vi "read1Byte Tx Rx.vi"(7 "address":u16, 8 "error in (no error)":errorcluster, 9 "id":u8, 10 "protocol_version":i32, 11 "port_num":i32) -> (0 "error out":errorcluster, 3 "function return":u8)   [LabVIEW 2018, in "labview.lvlib"]
doc: "WINDECLSPEC uint8_t read1ByteTxRx (int port_num, int protocol_version, uint8_t id, uint16_t address);"
uses:
  labview.lvlib
  dxl_x86_c.dll
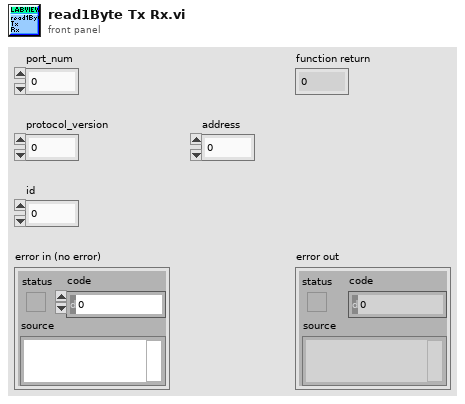
[diagram p1: front panel]
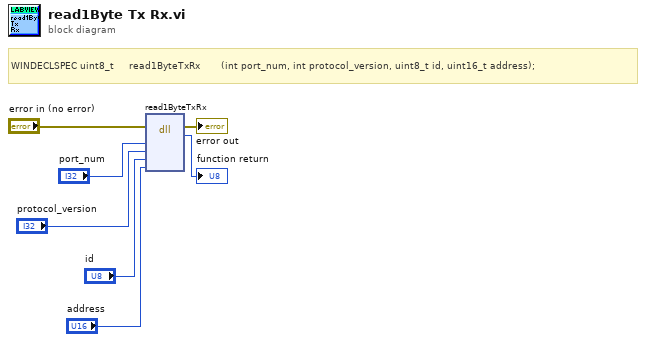
[diagram p0: block diagram]
diagram:
  # "WINDECLSPEC uint8_t     read1ByteTxRx       (int port_num, int protocol_version, uint8_t id, uint16_t address);"
  n1 = dll-call lib="C:/Users/joaos/OneDrive/Documents/[PhD]/Project Omnidirectional Vehicle/Vanes/LabView_code/joaoandthethreestands/DynamixelSDK-3.7.31/labview/new_compilation/dxl_x86_c.*" fn="read1ByteTxRx"(error in="error in (no error)", "port_num"="port_num", "protocol_version"="protocol_version", "id"="id", "address"="address") -> (error out=→"error out":errorcluster, →"function return":u8)  [unwired: 6 in, 1 out]
